vi "GUI_Bella_Triggers.vi"() -> ()   [LabVIEW 2020]
uses:
  Shared/GUI_Template/GUI_master/tcp_new_data_event.ctl
  Shared/GUI_Template/GUI_master/tcp new data cluster.ctl
panel:
  in  "trigger::32":bool=TRUE caption="Blank Button"
  in  "GUIdevice 32":string="CAM-LT-Tel4b"
  in  "Trigger.mode::29":u16(ring)=2 caption="Trigger mode" items=["Auto", "Normal", "Single", "Single, auto trigger"]
  in  "Trigger.Slope::29":u16(ring) caption="Trigger Slope" items=["Rising", "Falling"]
  in  "Trigger.Source::29":u16(ring)=1 caption="Trigger Source" items=["Channel 1", "Channel 2", "Channel 3", "Channel 4", "External", "Power Line"]
  in  "Trigger.Level::29":dbl=0.04 caption="Trigger Level (V)" min=0.0001 max=30.0 format="%#_6p"
  in  "Trigger.Mode::26":u16(ring) caption="Mode" items=["Immediate", "Analog Edge", "Analog Window", "Analog Hysteresis", "Video", "Digital Edge"]
  in  "Trigger.Mode::24":u16(ring) caption="Mode" items=["Immediate", "Analog Edge", "Analog Window", "Analog Hysteresis", "Video", "Digital Edge"]
  in  "Trigger.Mode::22":u16(ring) caption="Mode" items=["Immediate", "Analog Edge", "Analog Window", "Analog Hysteresis", "Video", "Digital Edge"]
  in  "trigger::31":bool=TRUE caption="Blank Button"
  in  "trigger::30":bool=TRUE caption="Blank Button"
  in  "trigger::21":bool=TRUE caption="Blank Button"
  in  "trigger::20":bool=TRUE caption="Blank Button"
  in  "trigger::19":bool=TRUE caption="Blank Button"
  in  "trigger::18":bool=TRUE caption="Blank Button"
  in  "trigger::16":bool=TRUE caption="Blank Button"
  in  "trigger::15":bool=TRUE caption="Blank Button"
  in  "trigger::14":bool=TRUE caption="Blank Button"
  in  "trigger::13":bool=TRUE caption="Blank Button"
  in  "trigger::12":bool=TRUE caption="Blank Button"
  in  "trigger::11":bool=TRUE caption="Blank Button"
  in  "trigger::10":bool=TRUE caption="Blank Button"
  in  "trigger::9":bool=TRUE caption="Blank Button"
  in  "trigger::7":bool=TRUE caption="Blank Button"
  in  "trigger::6":bool=TRUE caption="Blank Button"
  in  "trigger::5":bool=TRUE caption="Blank Button"
  in  "trigger::4":bool=TRUE caption="Blank Button"
  in  "trigger::3":bool=TRUE caption="Blank Button"
  in  "trigger::2":bool=TRUE caption="Blank Button"
  in  "trigger::1":bool=TRUE caption="Blank Button"
  in  "GUIdevice 31":string="SPEC-TEA-Qred"
  in  "GUIdevice 30":string="SPEC-AA-Hamamastsu"
  in  "Jet trigger":bool caption="Triggers"
  in  "GUIdevice 4":string="CAM-HPD-CCD"
  in  "GUIdevice 6":string="CAM-HPD-HolyWedge"
  in  "GUIdevice 29":string="SCOPE-AA-LeCroy8254M"
  in  "GUIdevice 26":string="DAQ-AA-3"
  in  "GUIdevice 24":string="DAQ-AA-2"
  in  "GUIdevice 22":string="DAQ-AA-1"
  in  "GUIdevice 21":string="CAM-TEA-MagSpecL"
  in  "GUIdevice 20":string="CAM-TEA-MagSpecK"
  in  "GUIdevice 19":string="CAM-TEA-MagSpecJ"
  in  "GUIdevice 18":string="CAM-TEA-MagSpecI"
  in  "GUIdevice 16":string="CAM-TEA-MagSpecH"
  in  "GUIdevice 15":string="CAM-TEA-MagSpecG"
  out "error IO 2":errorcluster
  out "tcp data event":T1
  in  "GUIdevice 14":string="CAM-TEA-MagSpecD"
  in  "GUIdevice 13":string="CAM-TEA-MagSpecC"
  in  "GUIdevice 7":string="CAM-PL1-APLSideView"
  in  "GUIdevice 2":string="CAM-1BL-M2"
  in  "GUIdevice 10":string="CAM-TEA-EBeam_Profile"
  in  "GUIdevice 5":string="CAM-HPD-HeatCCD"
  in  "GUIdevice 1":string="CAM-1BL-M1"
  in  "GUIdevice 3":string="CAM-1BL-M5"
  in  "GUIdevice 11":string="CAM-TEA-MagSpecA"
  in  "GUIdevice 12":string="CAM-TEA-MagSpecB"
  in  "GUIdevice 9":string="CAM-PL1-SideSpec"
  in  "stop":bool
  # "CAM-1BL-CompG4\n\nCAM-1BL-M1back\n\n\n\nCAM-2BL-GHOST\n\n\n\nCAM-HPD-CCD2\nCAM-HPD-CCD3\n\nCAM-HPD-HeatM3\n\n\nCAM-LT-SPLIT\nCAM-LT-XPW\n\nCAM-PL1-LPMode\nCAM-PL1-PMReflect\n\nCAM-PL1-SideSpec\nCAM-PL1-SideView\nCAM-PL1-TopView\n\n\n\n\n\n\n\n\nCAM-TEA-MagSpecHR\n\n\n\n\n\n\n\nEM-HPD-1\nEM-LB-1\nEM-LB-1\nEM-LB-PL\nFROG-HPD-1\nFROG-LB-1\nHPD-Phasics151\nIP2-MCPcam\nIP2-modeim\nIP2-Reflected1\nIP2-Reflected1\nIP2-targetobs\nIP2-targetscatt\nIP2-transmit\nP2-AndorCam\nP2-DG535\nP2-HeatCamPost\nP2-HeatCamPostNear\nP2-HeatCamPreFar\nP2-HeatCamPreNear\nP2-HeatCamPreNear\nP2-HeatEnergy\nP2-HeatEnergy\nP2-phasics\nP2-phasicsHR\nP2-ProbeCamPost\nP2-ProbeCamPostNear\nP2-ProbeCamPreNear\nP2-SideView\nP2-SRS\nP2-SRS\nP2FastDiag645\nP2FastDiag645\n\nSCOPE-LT-LeCroy64Xi\nSCOPE-PL1-PXIfast\nSCOPE-PL1-PXIfast\nSCOPE-PL1-PXIfast\nSCOPE-PL1-PXIfast\nSPEC-AA-Hamamastsu\nSPEC-PL1-Thorlabs\nSPEC-TEA-Qred"
  # "BELLA Triggers"
  # "Trigger"
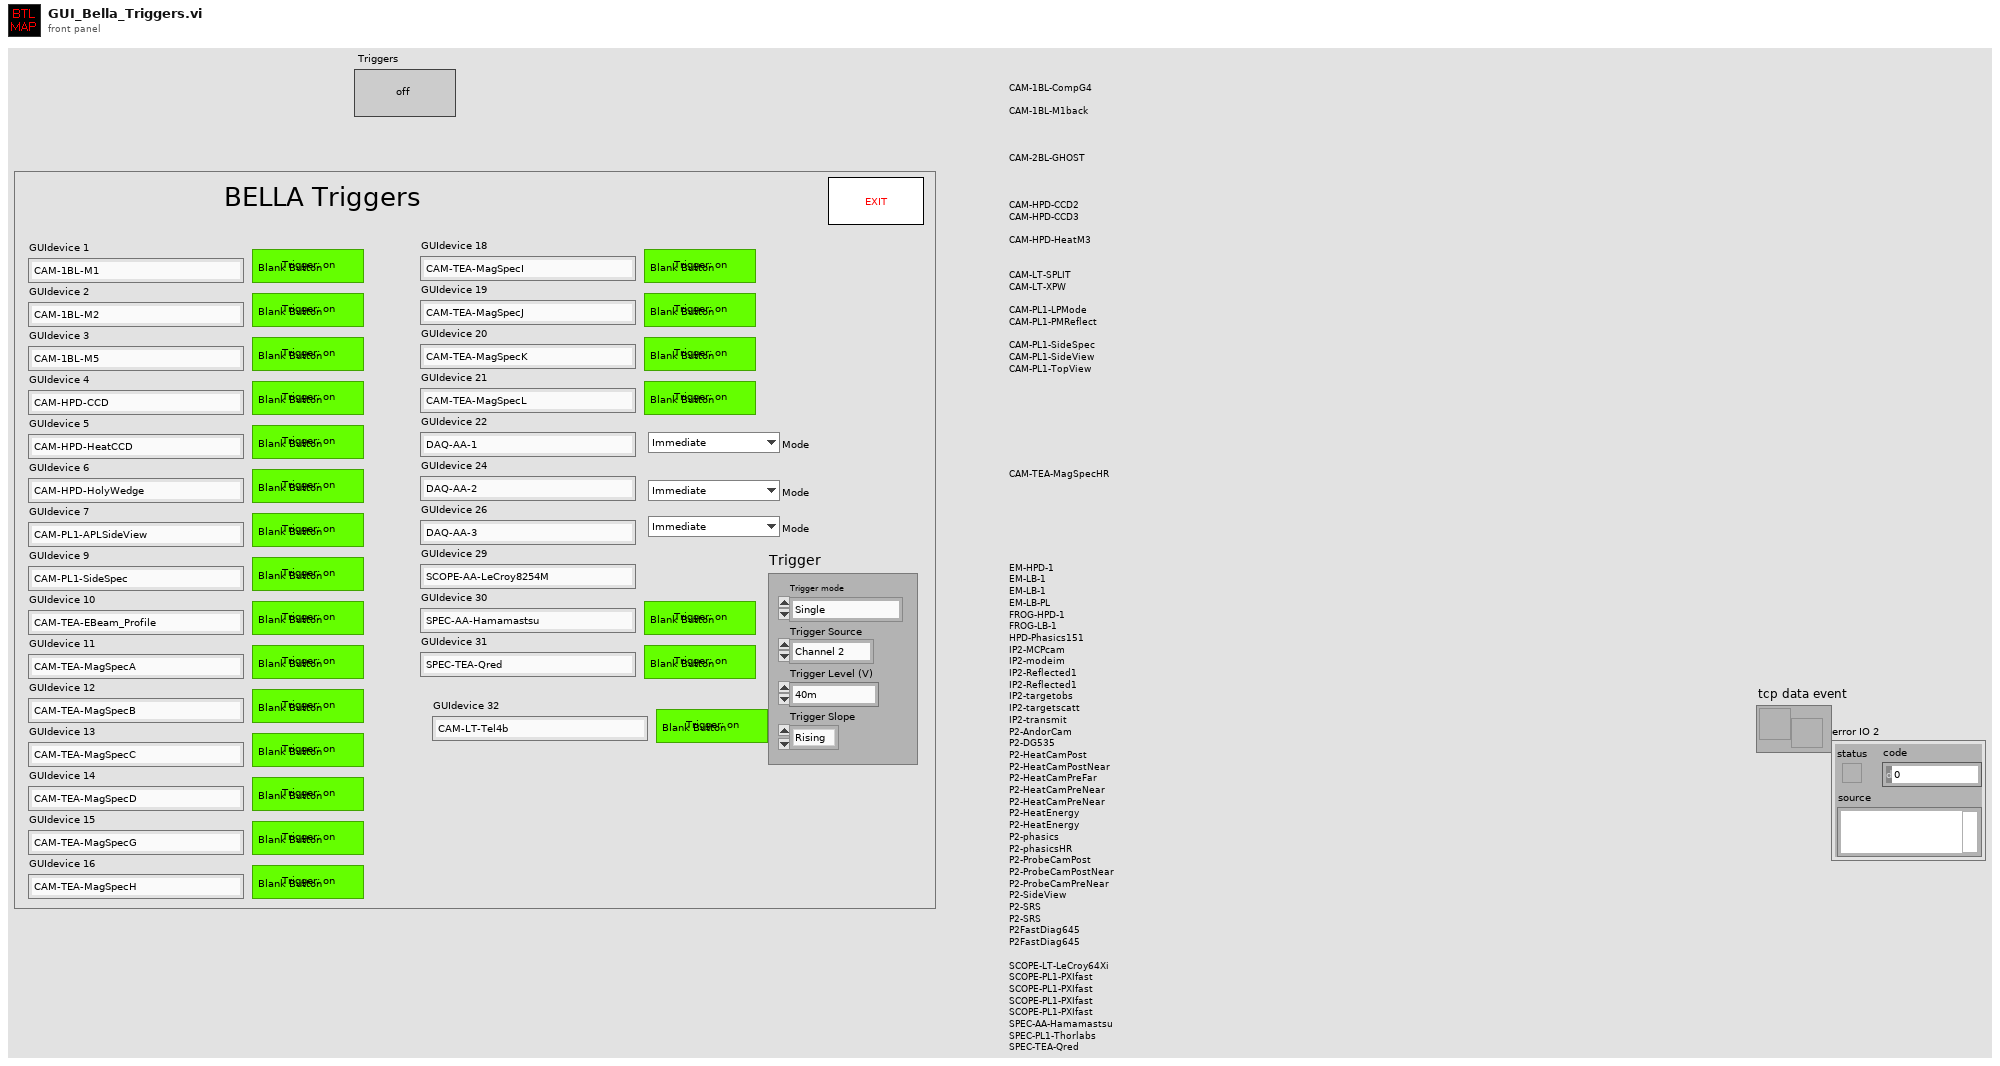
[diagram p1: front panel]
types:
  T1 = typedef "tcp_new_data_event.ctl" = refnum<user-event>
  T2 = typedef "tcp new data cluster.ctl" = cluster{"EventEnum":enum16{"new data", "connection status update"}, "Device name":string}
  T3 = enum32{"invalid app kind", "Development System", "Run Time System", "Student Edition", "Embedded LabVIEW", "Evaluation", "Custom"}
  T4 = enum32{"Invalid", "Standard", "Closed", "Hidden", "Minimized", "Maximized"}
  T5 = cluster{"Core":cluster{"Current VI Reference":refnum<vi>, "Close Panel on Exit?":bool}, "Heater timing offset":dbl, "Discharge timing offset":dbl, "Jet trigger":bool, "Tik1":u32, "Tik2":u32, "Fire Continues Allowed":bool}
  T6 = cluster{"Current VI Reference":refnum<vi>, "Close Panel on Exit?":bool}
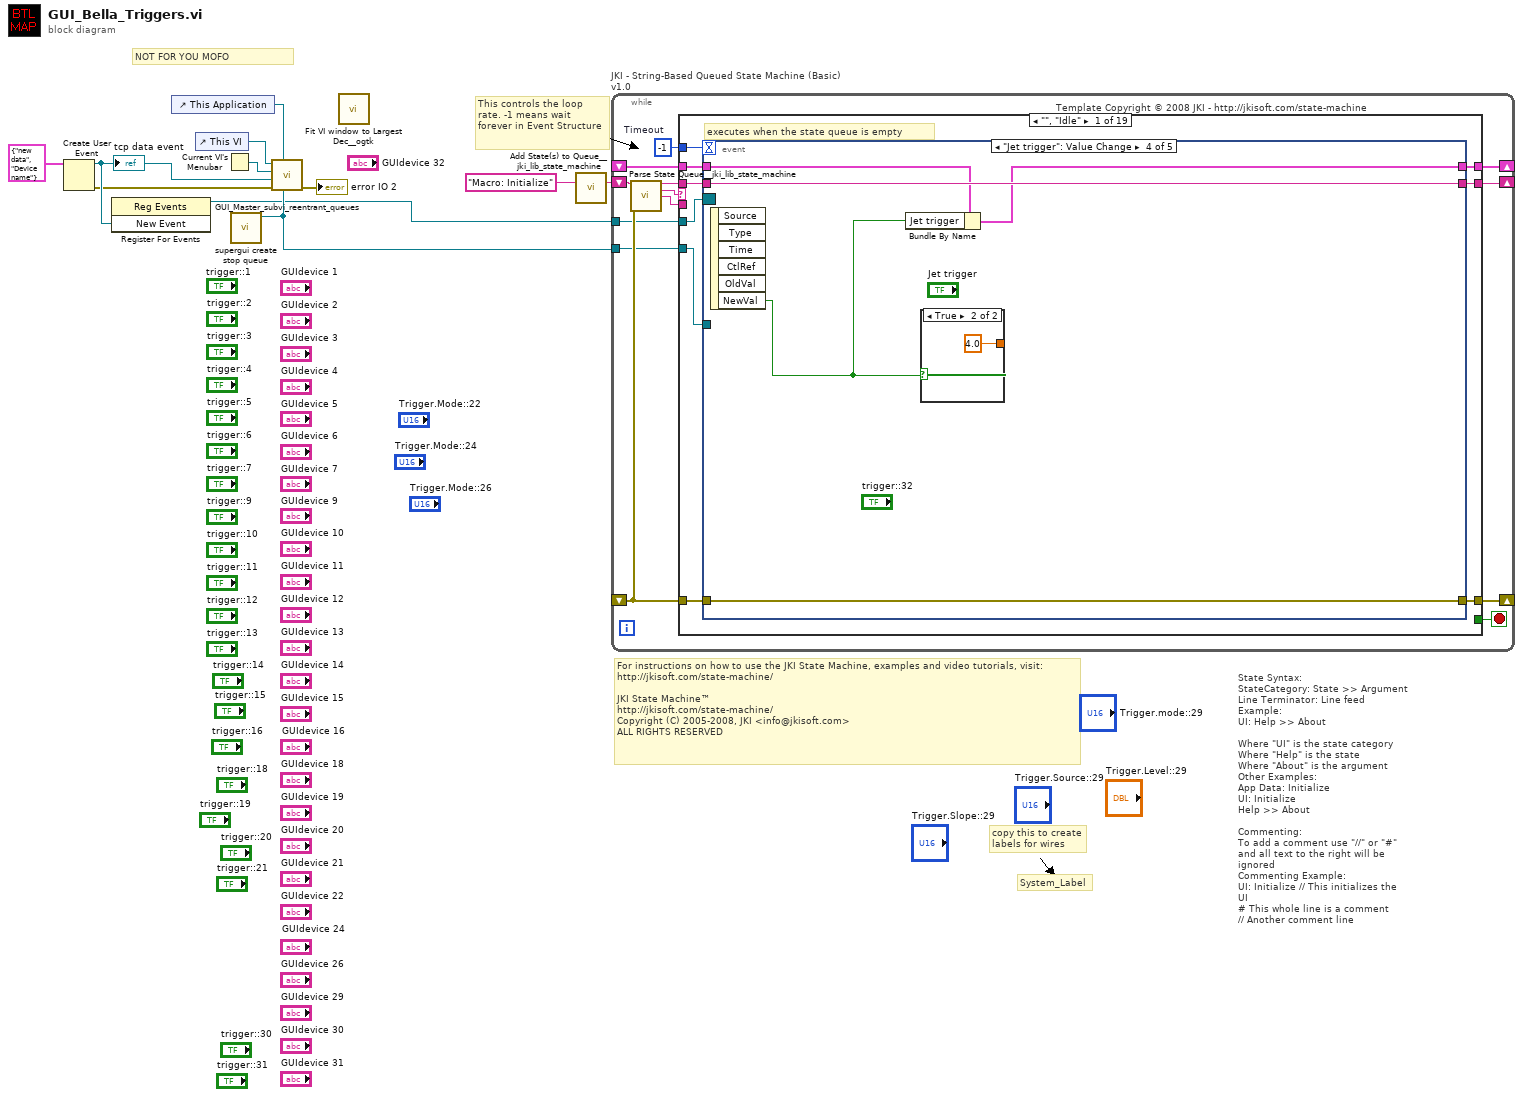
[diagram p0: block diagram]
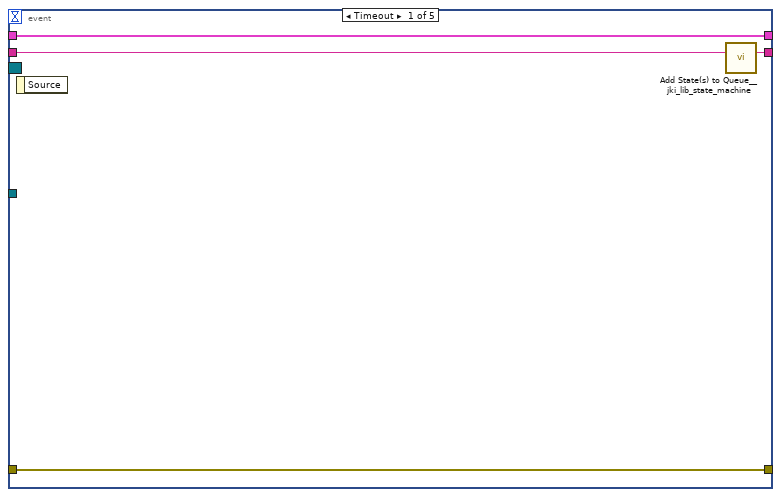
[diagram p2: hidden frame]
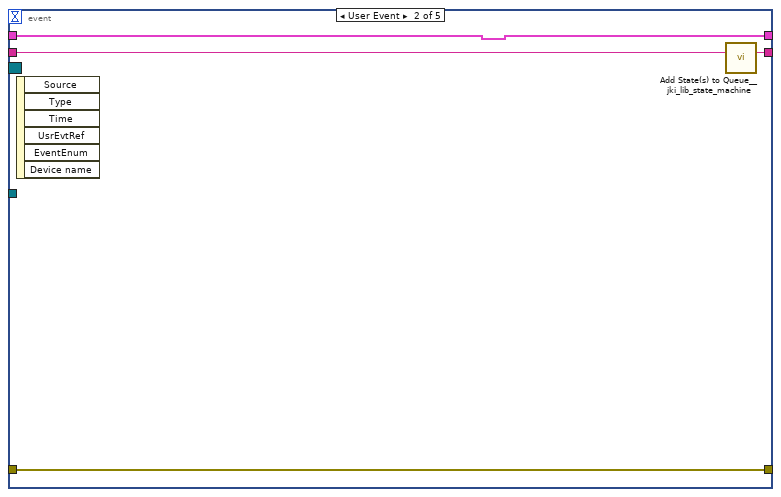
[diagram p3: hidden frame]
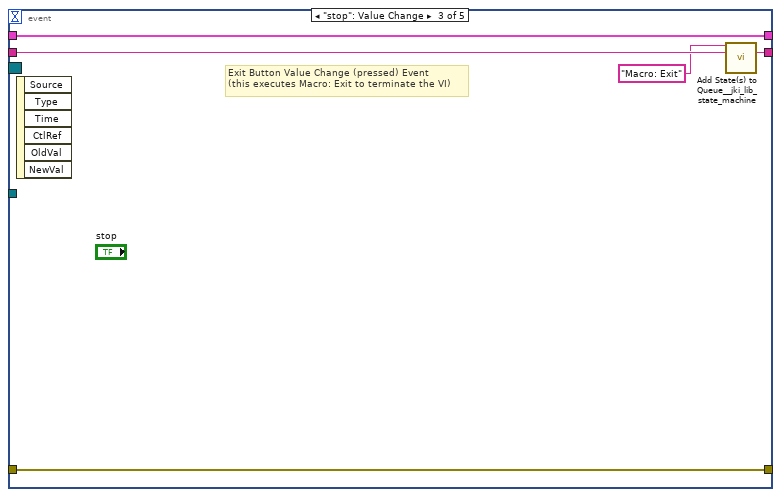
[diagram p4: hidden frame]
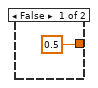
[diagram p5: hidden frame]
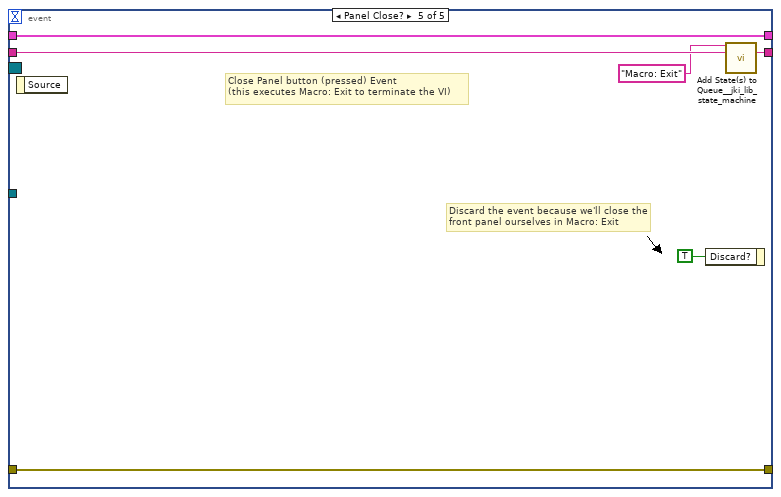
[diagram p6: hidden frame]
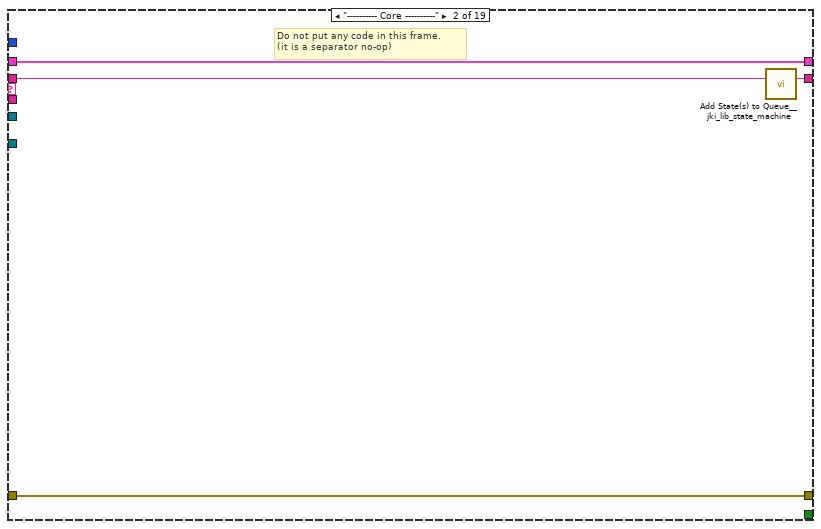
[diagram p7: hidden frame]
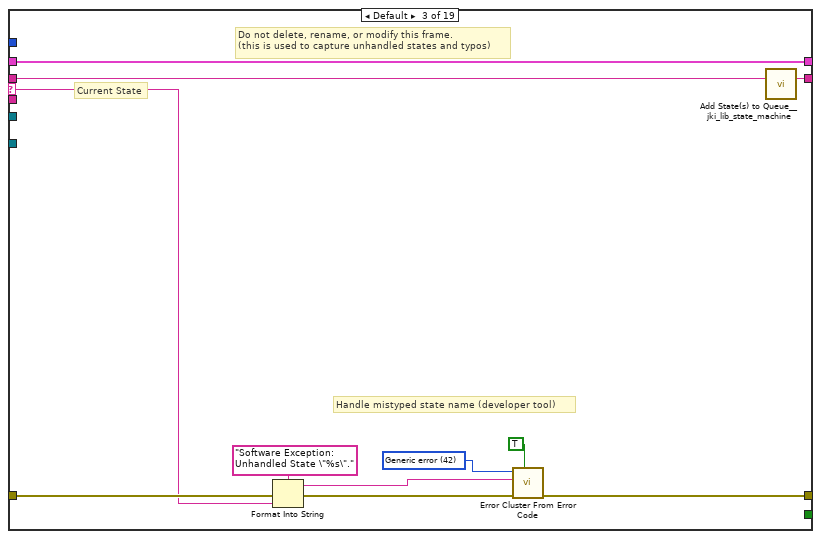
[diagram p8: hidden frame]
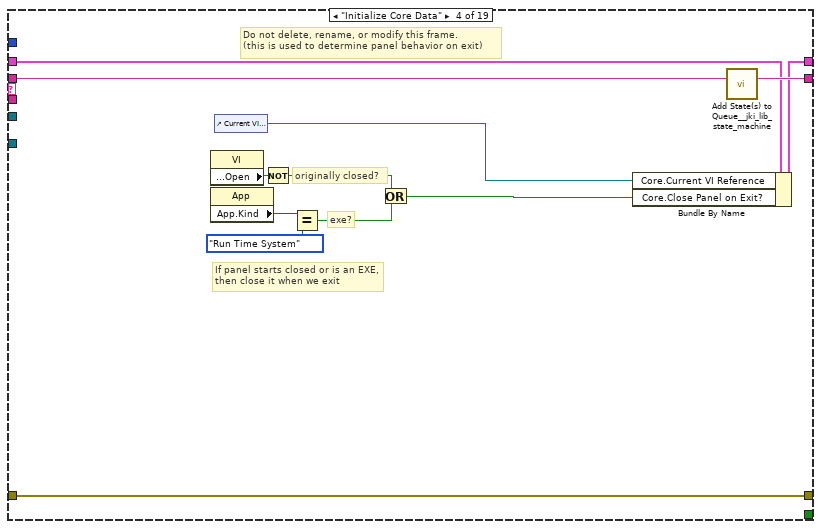
[diagram p9: hidden frame]
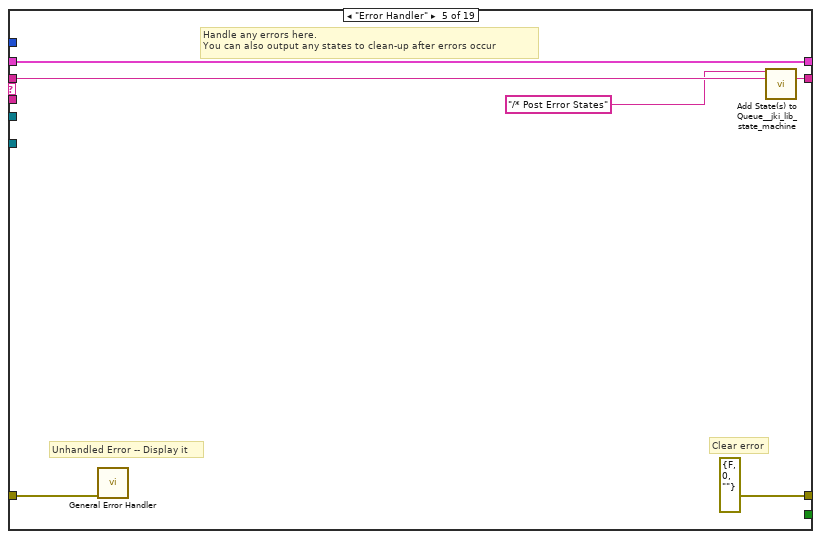
[diagram p10: hidden frame]
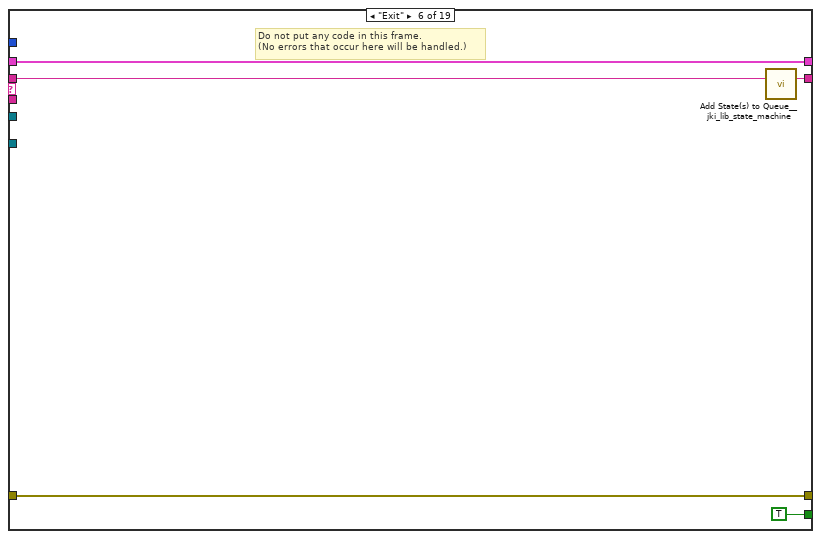
[diagram p11: hidden frame]
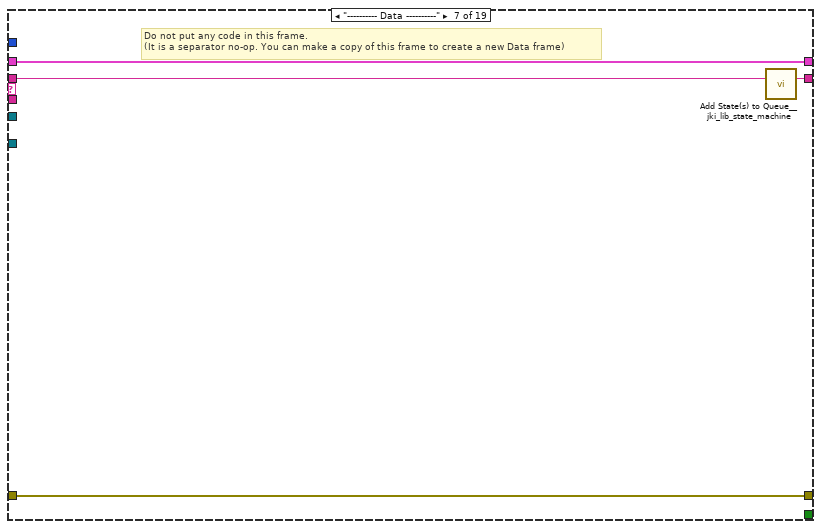
[diagram p12: hidden frame]
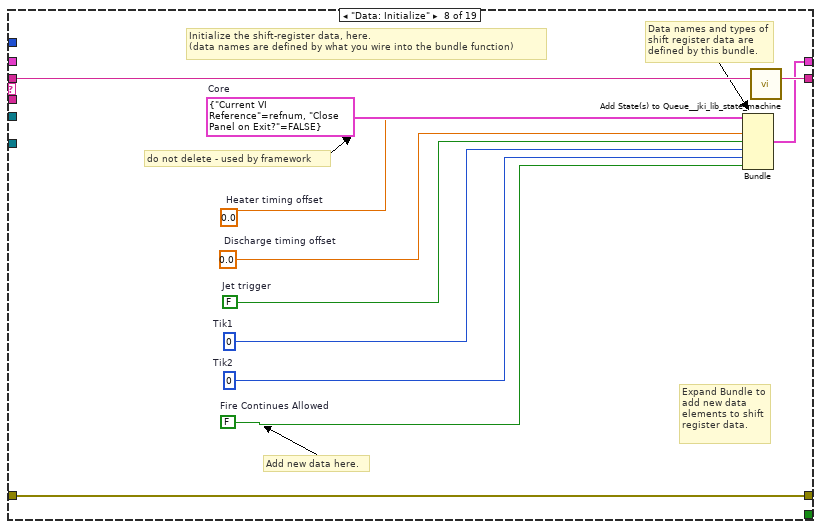
[diagram p13: hidden frame]
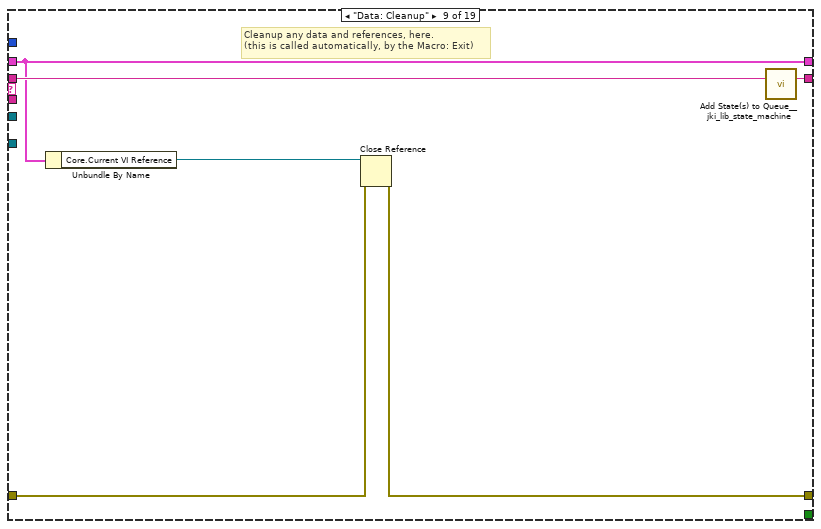
[diagram p14: hidden frame]
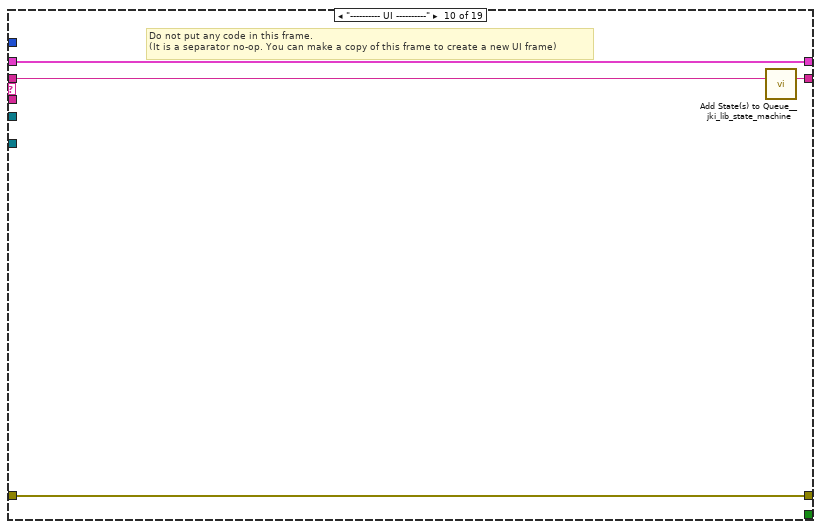
[diagram p15: hidden frame]
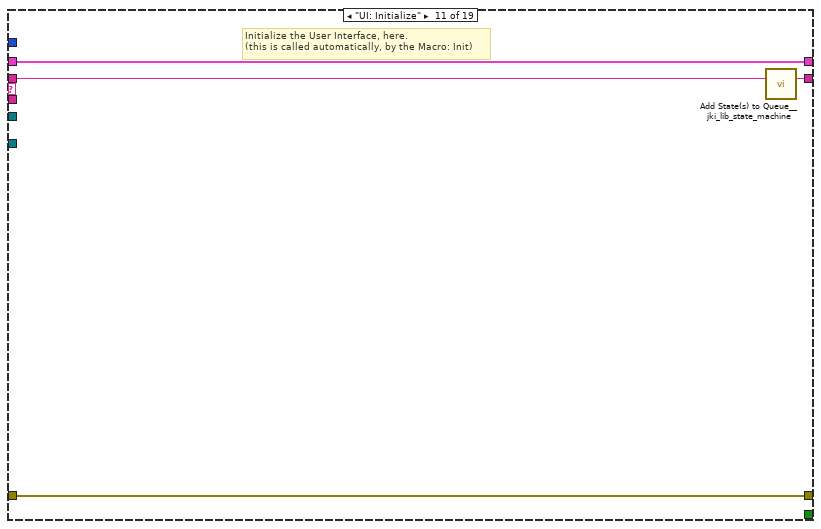
[diagram p16: hidden frame]
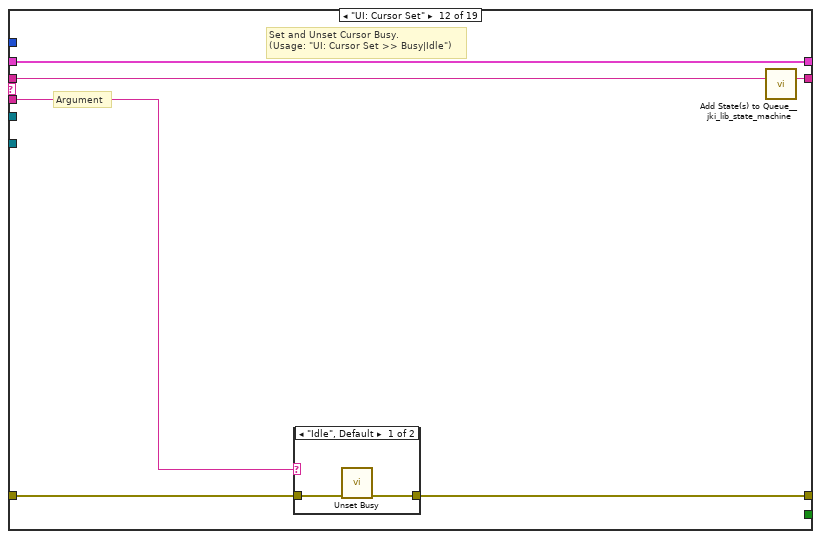
[diagram p17: hidden frame]
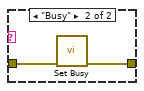
[diagram p18: hidden frame]
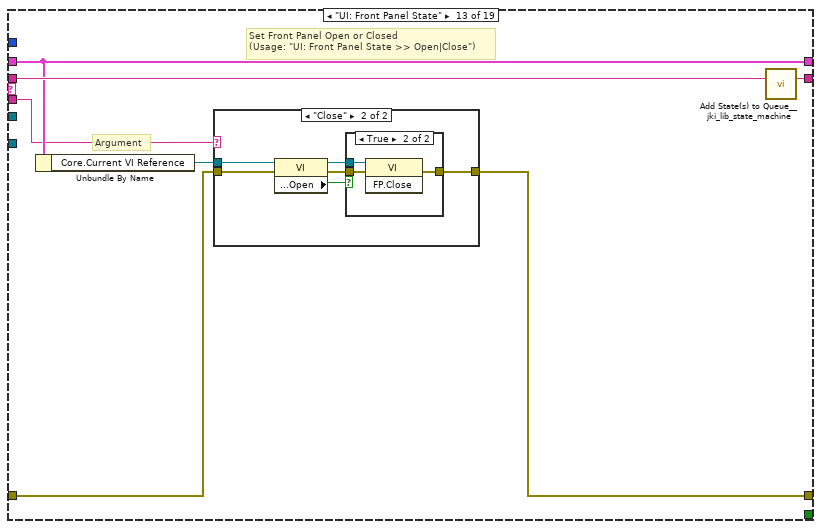
[diagram p19: hidden frame]
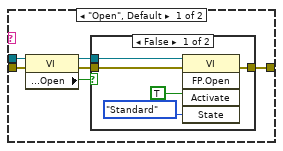
[diagram p20: hidden frame]
diagram:
  # "For instructions on how to use the JKI State Machine, examples and video tutorials, visit:\nhttp://jkisoft.com/state-machine/\n\nJKI State Machine™\nhttp://jkisoft.com/state-machine/\nCopyright (C) 2005-2008, JKI <info@jkisoft.com>\nALL RIGHTS RESERVED"
  # "State Syntax:\nStateCategory: State >> Argument\nLine Terminator: Line feed\nExample:\nUI: Help >> About\n\nWhere \"UI\" is the state category\nWhere \"Help\" is the state\nWhere \"About\" is the argument\nOther Examples:\nApp Data: Initialize\nUI: Initialize\nHelp >> About\n\nCommenting:\nTo add a comment use \"//\" or \"#\" and all text to the right will be ignored\nCommenting Example:\nUI: Initialize // This initializes the UI\n# This whole line is a comment\n// Another comment line"
  # "copy this to create labels for wires"
  # "This controls the loop rate. -1 means wait forever in Event Structure"
  # "System_Label"
  # "NOT FOR YOU MOFO"
  n1 = Create User Event(user event datatype=T2 {"EventEnum"=enum."new data", "Device name"="Device name"} ("New Event")) -> (user event=w10:refnum<user-event>, error out=w9:errorcluster)  [unwired: 1 in]
  "tcp data event" <- w10
  n2 = register-events(w10) -> (reference out=w1:refnum<event-registration>)  [unwired: 2 in, 1 out]
  n3 = control-ref of="This Application"() -> (w11:refnum<vi>)
  n4 = control-ref of="This VI"() -> (w5:refnum<vi>)
  n5 = Current VI's Menubar() -> (w7:refnum<k9>)
  n6 = call "supergui create stop queue.vi"() -> ("STOP Queue out"=w2:refnum<queue>)  [unwired: 11 in]
  n7 = call "GUI_Master_subvi_reentrant_queues.vi"("STOP Queue in"=w2, "This Application"=w11, "error in (no error)"=w9, "tcp data event"=w10, "Caller menu reference"=w7, "Caller VI ref"=w5) -> ("error out"=→"error IO 2":errorcluster)  [unwired: 5 in]
  n8 = call <userlib>:"Fit VI window to Largest Dec__ogtk.vi"() -> ()  [unwired: 6 in, 2 out]
  n9 = call <vilib>:"Add State(s) to Queue__jki_lib_state_machine.vi"("State(s) in (\"\")"="Macro: Initialize") -> ("States Out"=w3:string)  [unwired: 14 in]
  n10 = while "JKI - String-Based Queued State Machine (Basic) v1.0" {
    shift-right: [w17] -> _
    shift-left: _ -> [w16]
    shift-right: [w20] -> _
    shift-left: _ -> [w14]
    shift-right: [w19] -> _
    shift-left: w3 -> [w21]
    tunnel: w1 -> [w13]
    tunnel: w2 -> [w12]
    stop <- w18 stop-if-true
    w15 = -1  # Timeout
    # "Template Copyright © 2008 JKI - http://jkisoft.com/state-machine"
    n11 = call <vilib>:"Parse State Queue__jki_lib_state_machine.vi"("State Queue"=w21, "Error In (no error)"=w14) -> ("Remaining States"=w23:string, "Current State"=w24:string, "Arguments"=w22:string)  [unwired: 11 in]
    n12 = case shown="\"\", \"Idle\"" w24 {
      selector: w24 -> [_ _ w64 _ _ _ _ _ _ _ _ _ _ _ _ _ _ _ _]
      tunnel: w23 -> [w33 w63 w68 w86 w92 w97 w101 w112 w118 w122 w126 w132 w143 w169 w174 w187 w191 w203 w210]
      tunnel: w22 -> [_ _ _ _ _ _ _ _ _ _ _ w127 w137 _ _ _ _ _ _]
      tunnel: w16 -> [w31 w60 w66 w77 w89 w95 w98 _ w113 w119 w124 w130 w139 w166 w171 w184 w188 w200 w208]
      tunnel: [w30 w61 w70 w83 errorcluster {"status"=FALSE, "code"=0, "source"=""} ("error out") w94 w99 w109 w114 w120 w123 w128 w140 w167 w172 w185 w189 w201 w207] -> w20
      tunnel: w14 -> [w29 w61 w69 w83 w88 w94 w99 w109 w115 w120 w123 w129 w141 w167 w172 w185 w189 w201 w207]
      tunnel: [w32 w62 w67 w85 w91 w96 w100 w111 w117 w121 w125 w131 w142 w168 w173 w186 w190 w202 w209] -> w19
      tunnel: [_ _ _ _ _ TRUE _ _ _ _ _ _ _ _ _ _ _ _ _] -> w18
      tunnel: [w25 w60 w66 w84 w89 w95 w98 w110 w113 w119 w124 w130 w139 w166 w171 w184 w188 w199 w208] -> w17
      tunnel: w15 -> [w28 _ _ _ _ _ _ _ _ _ _ _ _ _ _ _ _ _ _]
      tunnel: w13 -> [w27 _ _ _ _ _ _ _ _ _ _ _ _ _ _ _ _ _ _]
      tunnel: w12 -> [w26 _ _ _ _ _ _ _ _ _ _ _ _ _ _ w176 _ _ _]
      frame "", "Idle" {
        # "executes when the state queue is empty"
        n13 = event shown="[3] \"Jet trigger\": Value Change" {
          selector: w27 -> [_ _ _ _ _]
          dyn-events: _ -> [_ _ _ _ _]
          timeout: w28 -> [_ _ _ _ _]
          tunnel: w33 -> [w37 w41 w46 w51 w59]
          tunnel: [w36 w40 w45 w51 w58] -> w32
          tunnel: w31 -> [w34 w38 w43 w50 w56]
          tunnel: [w35 w39 w44 w47 w57] -> w30
          tunnel: w29 -> [w35 w39 w44 w47 w57]
          tunnel: [w34 w38 w43 w49 w56] -> w25
          tunnel: w26 -> [_ _ _ _ _]
          event Timeout {
            n14 = event-data() -> ()  [unwired: 1 in, 1 out]
            n15 = call <vilib>:"Add State(s) to Queue__jki_lib_state_machine.vi"("State(s) in (\"\")"=w37) -> ("States Out"=w36:string)  [unwired: 14 in]
          }
          event User Event {
            n16 = event-data() -> ()  [unwired: 1 in, 6 out]
            n17 = call <vilib>:"Add State(s) to Queue__jki_lib_state_machine.vi"("State(s) in (\"\")"=w41) -> ("States Out"=w40:string)  [unwired: 14 in]
          }
          event "stop": Value Change {
            # "Exit Button Value Change (pressed) Event\n(this executes Macro: Exit to terminate the VI)"
            n18 = event-data() -> ()  [unwired: 1 in, 6 out]
            n19 = call <vilib>:"Add State(s) to Queue__jki_lib_state_machine.vi"("State(s) in Front (\"\")"="Macro: Exit", "State(s) in (\"\")"=w46) -> ("States Out"=w45:string)  [unwired: 13 in]
          }
          event "Jet trigger": Value Change {
            n20 = event-data() -> ("NewVal"=w48:bool)  [unwired: 1 in, 5 out]
            n21 = Bundle By Name(cluster=w50, "Jet trigger"=w48) -> (w49:T5)
            n22 = case shown="True" w48 {
              tunnel: [0.5 ("Amplitude.Ch CD::10") 4.0 ("Amplitude.Ch CD::10")] -> _
              frame False {
              }
              frame True {
              }
            }
          }
          event Panel Close? {
            # "Discard the event because we'll close the front panel ourselves in Macro: Exit"
            # "Close Panel button (pressed) Event\n(this executes Macro: Exit to terminate the VI)"
            n23 = event-data() -> ()  [unwired: 1 in, 1 out]
            n24 = event-data("Discard?"=TRUE) -> ()  [unwired: 1 in, 1 out]
            n25 = call <vilib>:"Add State(s) to Queue__jki_lib_state_machine.vi"("State(s) in Front (\"\")"="Macro: Exit", "State(s) in (\"\")"=w59) -> ("States Out"=w58:string)  [unwired: 13 in]
          }
        }
      }
      frame "---------- Core ----------" {
        # "Do not put any code in this frame.\n(it is a separator no-op)"
        n26 = call <vilib>:"Add State(s) to Queue__jki_lib_state_machine.vi"("State(s) in (\"\")"=w63) -> ("States Out"=w62:string)  [unwired: 14 in]
      }
      frame Default {
        w73 = 42 items=["No error", "Argument error", "Memory is full", "Out of zone", "End of file", "File already open", "Generic file I/O error", "File not found", "File permission error", "Disk is full", "Duplicate path", "Too many files open", "System feature not enabled", "Resource file not found", "Cannot add resource", "Resource not found", "Image not found", "Image memory error", "Pen does not exist", "Config type invalid", "Config token not found", "Config parse error", "Config memory error", "Bad external code format", "Bad external code offset", "External code not present", "Null window", "Destroy window error", "Null menu", "Print aborted", "Bad print record", "Print driver error", "Windows error during printing", "Memory error during printing", "Print dialog error", "Generic print error", "Invalid device refnum", "Device not found", "Device parameter error", "Device unit error", "Cannot open device", "Device call aborted", "Generic error", "Cancelled by user", "Object ID too low", "Object ID too high", "Object not in heap", "Unknown heap", "Unknown object (invalid DefProc)", "Unknown object (DefProc not in table)", "Message out of range", "Invalid (null) method", "Unknown message", "Manager call not supported", "Bad address", "Network operation in progress", "Network operation timed out", "Connection is busy", "Network attribute not supported", "Network error", "Address in use", "System out of memory", "Connection aborted", "Connection refused", "Not connected", "Already connected", "Connection closed", "Initialization error (interapplication manager)", "Bad occurrence", "Wait on unbound occurrence handler", "Occurrence queue overflow", "Datalog type conflict", "Unused", "Unrecognized type (interapplication manager)", "Memory corrupt", "Failed to make temporary DLL", "Old CIN version", "Drag socket not found", "Failed to load drop-object", "Failed to register OLE object", "Failed to release OLE object", "Format specifier type mismatch", "Unknown format specifier", "Too few format specifiers", "Too many format specifiers", "Scan failed", "Newer CIN version", "Error converting to variant", "Runtime menu error", "Password tampered", "Variant attribute not found", "Incompatible variant data type", "Event data is not available", "Event Store is not present", "Occurrence is not found", "Event Queue is not created", "Event info is not available", "Refnum passed is NULL", "Error retrieving Class GUID", "Error retrieving CoClass GUID", "Error retrieving TypeLib GUID.", "Bad built application magic bytes.", "Specific driver is different from the specific driver associated with the Logical Name.", "There is no session opened to the class driver.", "Max Error", "MAX - Error with config objects", "MAX - Error loading configuration", "MAX - Group not supported"]
        # "Current State"
        # "Do not delete, rename, or modify this frame.\n(this is used to capture unhandled states and typos)"
        # "Handle mistyped state name (developer tool)"
        n27 = Format Into String(format string="Software Exception: Unhandled State \"%s\"." ("message"), error in=w69, w64) -> (resulting string=w72:string, error out=w71:errorcluster)  [unwired: 1 in]
        n28 = call <vilib>:"Error Cluster From Error Code.vi"("show call chain? (False)"=TRUE, "error in (no error)"=w71, "error message (\"\")"=w72, "error code (0)"=w73) -> ("error out"=w70:errorcluster)  [unwired: 5 in]
        n29 = call <vilib>:"Add State(s) to Queue__jki_lib_state_machine.vi"("State(s) in (\"\")"=w68) -> ("States Out"=w67:string)  [unwired: 14 in]
      }
      frame "Initialize Core Data" {
        # "Do not delete, rename, or modify this frame.\n(this is used to determine panel behavior on exit)"
        # "originally closed?"
        # "exe?"
        # "If panel starts closed or is an EXE, then close it when we exit"
        n30 = property class="VI"() -> ("Front Panel.Open"=w82:bool)  [unwired: 2 in, 2 out]
        n31 = property class="App"() -> ("App.Kind"=w81:T3)  [unwired: 2 in, 2 out]
        n32 = control-ref of="Current VI Reference"() -> (w75:refnum<vi>)
        n33 = Not(x=w82) -> (.not. x?=w79:bool)
        n34 = Equal?(x=w81, y=T3."Run Time System" ("Application:Kind")) -> (x = y?=w78:bool)
        n35 = Or(x=w79, y=w78) -> (x .or. y?=w76:bool)
        n36 = Bundle By Name(cluster=w77, "Core.Current VI Reference"=w75, "Core.Close Panel on Exit?"=w76) -> (w84:T5)
        n37 = call <vilib>:"Add State(s) to Queue__jki_lib_state_machine.vi"("State(s) in (\"\")"=w86) -> ("States Out"=w85:string)  [unwired: 14 in]
      }
      frame "Error Handler" {
        # "Unhandled Error -- Display it"
        # "Handle any errors here.\nYou can also output any states to clean-up after errors occur"
        # "Clear error"
        n38 = call <vilib>:"General Error Handler.vi"("error in (no error)"=w88) -> ()  [unwired: 10 in, 5 out]
        n39 = call <vilib>:"Add State(s) to Queue__jki_lib_state_machine.vi"("State(s) in Front (\"\")"="/* Post Error States", "State(s) in (\"\")"=w92) -> ("States Out"=w91:string)  [unwired: 13 in]
      }
      frame "Exit" {
        # "Do not put any code in this frame.\n(No errors that occur here will be handled.)"
        n40 = call <vilib>:"Add State(s) to Queue__jki_lib_state_machine.vi"("State(s) in (\"\")"=w97) -> ("States Out"=w96:string)  [unwired: 14 in]
      }
      frame "---------- Data ----------" {
        # "Do not put any code in this frame.\n(It is a separator no-op. You can make a copy of this frame to create a new Data frame)"
        n41 = call <vilib>:"Add State(s) to Queue__jki_lib_state_machine.vi"("State(s) in (\"\")"=w101) -> ("States Out"=w100:string)  [unwired: 14 in]
      }
      frame "Data: Initialize" {
        w102 = FALSE  # Fire Continues Allowed
        w104 = u32 0  # Tik1
        w103 = u32 0  # Tik2
        w105 = FALSE  # Jet trigger
        w106 = 0.0  # Discharge timing offset
        w107 = 0.0  # Heater timing offset
        w108 = T6 {"Current VI Reference"=refnum, "Close Panel on Exit?"=FALSE}  # Core
        # "do not delete - used by framework"
        # "Expand Bundle to add new data elements to shift register data."
        # "Add new data here."
        # "Data names and types of shift register data are defined by this bundle."
        # "Initialize the shift-register data, here.\n(data names are defined by what you wire into the bundle function)"
        n42 = Bundle("Core"=w108, "Heater timing offset"=w107, "Discharge timing offset"=w106, "Jet trigger"=w105, "Tik1"=w104, "Tik2"=w103, "Fire Continues Allowed"=w102) -> (w110:T5)  [unwired: 1 in]
        n43 = call <vilib>:"Add State(s) to Queue__jki_lib_state_machine.vi"("State(s) in (\"\")"=w112) -> ("States Out"=w111:string)  [unwired: 14 in]
      }
      frame "Data: Cleanup" {
        # "Cleanup any data and references, here.\n(this is called automatically, by the Macro: Exit)"
        n44 = Unbundle By Name(w113) -> ("Core.Current VI Reference"=w116:refnum<vi>)
        n45 = Close Reference(reference=w116, error in (no error)=w115) -> (error out=w114:errorcluster)
        n46 = call <vilib>:"Add State(s) to Queue__jki_lib_state_machine.vi"("State(s) in (\"\")"=w118) -> ("States Out"=w117:string)  [unwired: 14 in]
      }
      frame "---------- UI ----------" {
        # "Do not put any code in this frame.\n(It is a separator no-op. You can make a copy of this frame to create a new UI frame)"
        n47 = call <vilib>:"Add State(s) to Queue__jki_lib_state_machine.vi"("State(s) in (\"\")"=w122) -> ("States Out"=w121:string)  [unwired: 14 in]
      }
      frame "UI: Initialize" {
        # "Initialize the User Interface, here.\n(this is called automatically, by the Macro: Init)"
        n48 = call <vilib>:"Add State(s) to Queue__jki_lib_state_machine.vi"("State(s) in (\"\")"=w126) -> ("States Out"=w125:string)  [unwired: 14 in]
      }
      frame "UI: Cursor Set" {
        # "Argument"
        # "Set and Unset Cursor Busy.\n(Usage: \"UI: Cursor Set >> Busy|Idle\")"
        n49 = case shown="\"Idle\", Default" w127 {
          tunnel: w129 -> [w134 w136]
          tunnel: [w133 w135] -> w128
          frame "Idle", Default {
            n50 = call <vilib>:"Unset Busy.vi"("error in (no error)"=w134) -> ("error out"=w133:errorcluster)  [unwired: 10 in]
          }
          frame "Busy" {
            n51 = call <vilib>:"Set Busy.vi"("error in (no error)"=w136) -> ("error out"=w135:errorcluster)  [unwired: 9 in, 1 out]
          }
        }
        n52 = call <vilib>:"Add State(s) to Queue__jki_lib_state_machine.vi"("State(s) in (\"\")"=w132) -> ("States Out"=w131:string)  [unwired: 14 in]
      }
      frame "UI: Front Panel State" {
        # "Argument"
        # "Set Front Panel Open or Closed\n(Usage: \"UI: Front Panel State >> Open|Close\")"
        n53 = Unbundle By Name(w139) -> ("Core.Current VI Reference"=w138:refnum<vi>)
        n54 = case shown="\"Close\"" w137 {
          tunnel: w141 -> [w147 w160]
          tunnel: [w149 w161] -> w140
          tunnel: w138 -> [w148 w158]
          frame "Open", Default {
            n55 = property class="VI"(reference=w148, error in=w147) -> (reference out=w145:refnum<vi>, error out=w146:errorcluster, "Front Panel.Open"=w144:bool)
            n56 = case shown="False" w144 {
              tunnel: [w152 w155] -> w149
              tunnel: w146 -> [w151 w155]
              tunnel: w145 -> [w150 _]
              frame False {
                n57 = invoke class="VI" method="FP.Open"(reference=w150, error in=w151, "Activate"=TRUE, "State"=T4."Standard") -> (error out=w152:errorcluster)  [unwired: 1 in, 4 out]
              }
              frame True {
              }
            }
          }
          frame "Close" {
            n58 = property class="VI"(reference=w158, error in=w160) -> (reference out=w157:refnum<vi>, error out=w159:errorcluster, "Front Panel.Open"=w156:bool)
            n59 = case shown="True" w156 {
              tunnel: [w162 w165] -> w161
              tunnel: w159 -> [w162 w164]
              tunnel: w157 -> [_ w163]
              frame False {
              }
              frame True {
                n60 = invoke class="VI" method="FP.Close"(reference=w163, error in=w164) -> (error out=w165:errorcluster)  [unwired: 1 in, 2 out]
              }
            }
          }
        }
        n61 = call <vilib>:"Add State(s) to Queue__jki_lib_state_machine.vi"("State(s) in (\"\")"=w143) -> ("States Out"=w142:string)  [unwired: 14 in]
      }
      frame "---------- Macro ----------" {
        # "Do not put any code in this frame.\n(It is a separator no-op. You can make a copy of this frame to create a new Macro frame)"
        n62 = call <vilib>:"Add State(s) to Queue__jki_lib_state_machine.vi"("State(s) in (\"\")"=w169) -> ("States Out"=w168:string)  [unwired: 14 in]
      }
      frame "Macro: Initialize" {
        # "Initialization Macro\n(This is called once, when the VI starts)"
        n63 = call <vilib>:"Add State(s) to Queue__jki_lib_state_machine.vi"("State(s) in Front (\"\")"="Data: Initialize\nInitialize Core Data\nUI: Initialize\nUI: Front Panel State >> Open", "State(s) in (\"\")"=w174) -> ("States Out"=w173:string)  [unwired: 13 in]
      }
      frame "Macro: Exit" {
        # "Exit Macro\n(This is called once, when the VI exits)"
        n64 = Unbundle By Name(w184) -> ("Core.Close Panel on Exit?"=w183:bool)
        n65 = Release Queue(queue=w176, force destroy? (F)=TRUE) -> (error out=w175:errorcluster)  [unwired: 1 in, 2 out]
        n66 = call <vilib>:"Clear Errors.vi"("error in (no error)"=w175) -> ()  [unwired: 5 in, 2 out]
        n67 = Select(t="UI: Front Panel State >> Close", s=w183, f="") -> (s? t:f=w180:string)
        n68 = call <vilib>:"Add State(s) to Queue__jki_lib_state_machine.vi"("State(s) in (\"\")"=w180, "State(s) at Back (\"\")"="Data: Cleanup\nExit") -> ("States Out"=w178:string)  [unwired: 13 in]
        n69 = call <vilib>:"Add State(s) to Queue__jki_lib_state_machine.vi"("State(s) in Front (\"\")"=w178, "State(s) in (\"\")"=w187) -> ("States Out"=w186:string)  [unwired: 13 in]
      }
      frame "---------- New Category ----------" {
        # "Template Separator\n(You can make a copy of, or modify, this frame)"
        n70 = call <vilib>:"Add State(s) to Queue__jki_lib_state_machine.vi"("State(s) in (\"\")"=w191) -> ("States Out"=w190:string)  [unwired: 14 in]
      }
      frame "Obsolete" {
        # "Your code here.\n(You can make a copy of, or modify, this frame)"
        n71 = Unbundle By Name(w200) -> ("Tik2"=w193:u32)
        n72 = Tick Count (ms)() -> (millisecond timer value=w195:u32)
        n73 = Subtract(x=w195, y=w193) -> (x-y=w198:u32)
        n74 = Greater?(x=w198, y=2000) -> (0:w196:bool)
        n75 = case shown="True" w196 {
          tunnel: w195 -> [_ w206]
          tunnel: [w204 w206] -> w194
          tunnel: w193 -> [w204 _]
          tunnel: [_ ""] -> w192
          frame False {
          }
          frame True {
          }
        }
        n76 = Bundle By Name(cluster=w200, "Tik2"=w194) -> (w199:T5)
        n77 = call <vilib>:"Add State(s) to Queue__jki_lib_state_machine.vi"("State(s) in Front (\"\")"=w192, "State(s) in (\"\")"=w203) -> ("States Out"=w202:string)  [unwired: 13 in]
      }
      frame "Action: Trig on" {
        (unwired) "fire>>force" ("Value (Signaling)")
        n78 = call <vilib>:"Add State(s) to Queue__jki_lib_state_machine.vi"("State(s) in (\"\")"=w210) -> ("States Out"=w209:string)  [unwired: 14 in]
      }
    }
  }
